vi "Parameters_Get_Position.vi"(11 "Parameters":dbl[](array[numeric])) -> (0 "Acceleration Jerk":dbl=1000.0, 1 "Acceleration":dbl=10000.0, 2 "Velocity":dbl=1000.0, 3 "Target Position":dbl[](array[numeric]))   [LabVIEW 2017, in "WordManipulationLibrary.lvlib"]
uses:
  WordManipulationLibrary.lvlib
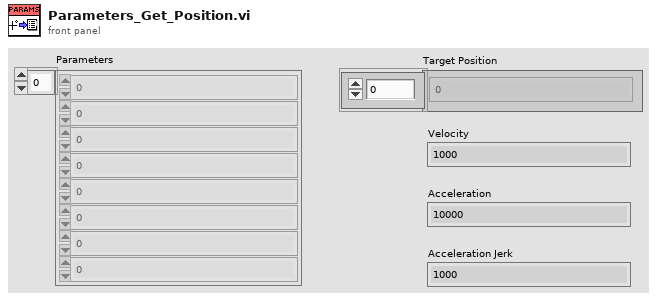
[diagram p1: front panel]
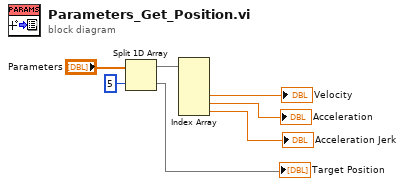
[diagram p0: block diagram]
diagram:
  n1 = Split 1D Array(array="Parameters", index=5) -> (first subarray=w2:dbl[], second subarray=→"Target Position":dbl[])
  n2 = Index Array(array=w2) -> (element #3=→"Velocity":dbl, element #4=→"Acceleration":dbl, element #5=→"Acceleration Jerk":dbl)  [unwired: 5 in, 2 out]
